vi "test Counter.vi"(8 "error in (no error)":errorcluster, 11 "TestCase in":refnum<class "Scan Engine Specialty Digital System Tests.lvclass">) -> (0 "error out":errorcluster, 3 "TestCase out":refnum<class "Scan Engine Specialty Digital System Tests.lvclass">)   [LabVIEW 2019, in "Scan Engine Specialty Digital System Tests.lvclass"]
uses:
  Scan Engine Specialty Digital System Tests.lvclass
  <vilib>/addons/_JKI Toolkits/VI Tester/TestCase.llb/TestCase.lvclass
  <vilib>/NI/VeriStand Custom Device Testing Tools/VeriStandTestUtilities/VeriStandTestUtilities.lvlib
  C:/Users/nitest/Desktop/Git 2019/niveristand-custom-device-testing-tools/VeriStandTestCase/VeriStandTestCase.lvclass
  C:/Program Files (x86)/National Instruments/LabVIEW 2019/vi.lib/addons/_JKI Toolkits/VI Tester/TestCase.llb/TestCase.lvclass
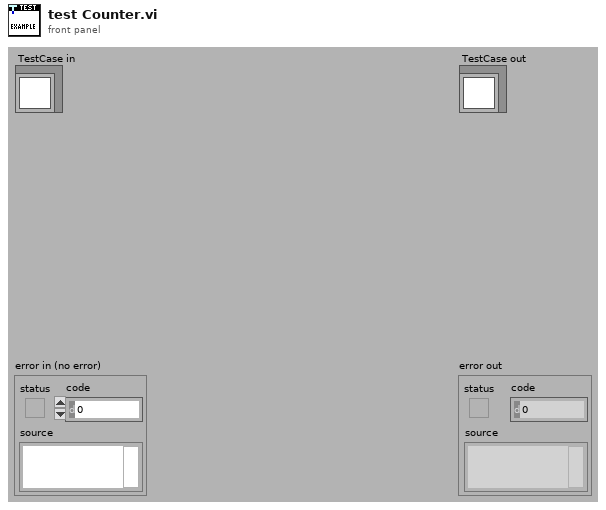
[diagram p1: front panel]
types:
  T1 = typedef "NI_VS Workspace ExecutionAPI.lvlib/WorkspaceAPI.ctl" = refnum<k24>
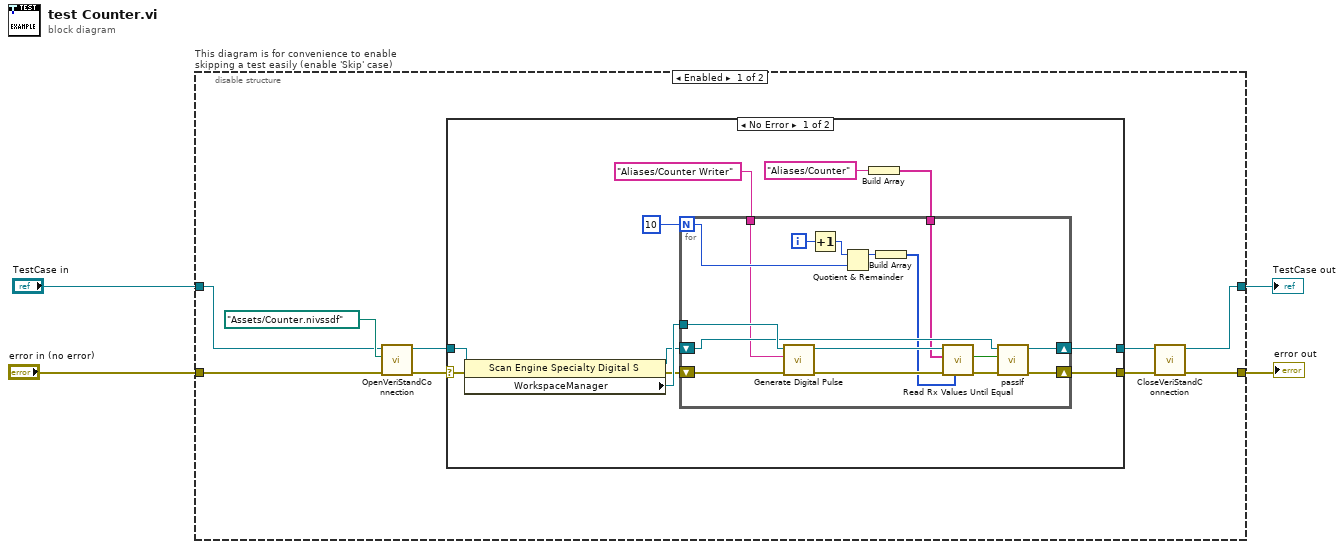
[diagram p0: block diagram]
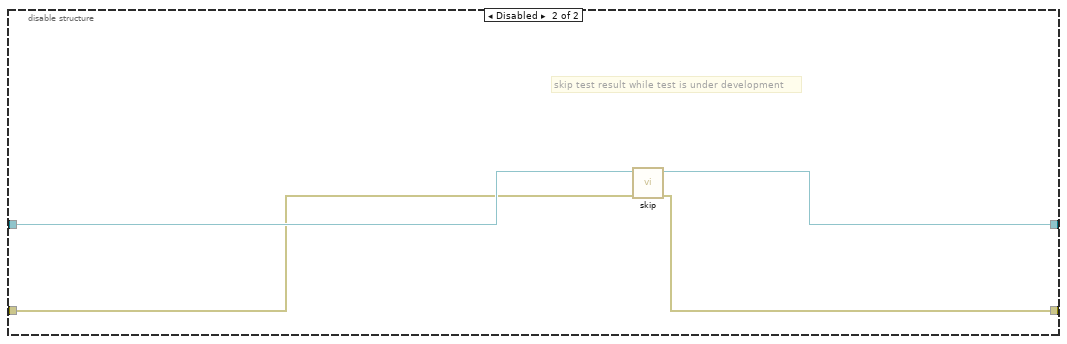
[diagram p3: hidden frame]
diagram:
  n1 = disable-structure "This diagram is for convenience to enable skipping a test easily (enable 'Skip' case)" shown="Enabled" {
    disable-tunnel: "TestCase in" -> [w9 w46]
    disable-tunnel: [w5 w44] -> w1
    disable-tunnel: [w7 w45] -> w3
    disable-tunnel: "error in (no error)" -> [w11 w43]
    frame Enabled {
      n2 = call-dynamic "OpenVeriStandConnection.vi"("error in (no error)"=w11, "System Definition File"=path "Assets/Counter.nivssdf", "VeriStand Test Case in"=w9) -> ("error out"=w12:errorcluster, "VeriStand Test Case out"=w10:refnum<class "Scan Engine Specialty Digital System Tests.lvclass">)  [unwired: 6 in, 1 out]
      n3 = case shown="No Error" w12 {
        selector: w12 -> [w17 w42]
        tunnel: [w21 w42] -> w8
        tunnel: [w15 w41] -> w6
        tunnel: w10 -> [w16 w41]
        frame No Error {
          n4 = property class="Scan Engine Specialty Digital S"(reference=w16, error in=w17) -> (reference out=w20:refnum<class "Scan Engine Specialty Digital System Tests.lvclass">, error out=w23:errorcluster, "WorkspaceManager"=w24:T1)
          n5 = Build Array("Aliases/Counter" ("Channel")) -> (w14:string[])
          n6 = for {
            N: 10 ("Terminal Count") -> [w30]
            tunnel: w24 -> [w40]
            shift-right: [w35] -> w21
            shift-left: w23 -> [w39]
            shift-right: [w32] -> w15
            shift-left: w20 -> [w33]
            tunnel: w14 -> [w28]
            tunnel: "Aliases/Counter Writer" ("Channel") -> [w29]
            i -> [w34]
            n7 = call "Generate Digital Pulse.vi"("error in (no error)"=w39, "Channel"=w29, "WorkspaceManager"=w40) -> ("error out"=w38:errorcluster, "Workspace Manager out"=w37:T1)  [unwired: 7 in]
            n8 = Increment(x=w34) -> (x+1=w31:i32)
            n9 = Quotient & Remainder(x=w31, y=w30) -> (x-y*floor(x/y)=w26:i32)  [unwired: 1 out]
            n10 = Build Array(w26) -> (w25:i32[])
            n11 = call <vilib>:"Read Rx Values Until Equal.vi"("expected values"=w25, "error in"=w38, "Rx aliases"=w28, "workspace manager in"=w37) -> ("error out"=w36:errorcluster, "values equal expected"=w27:bool)  [unwired: 5 in, 1 out]
            n12 = call-dynamic "passIf.vi"("error in (no error)"=w36, "pass"=w27, "TestCase in"=w33) -> ("error out"=w35:errorcluster, "TestCase out"=w32:refnum<class "Scan Engine Specialty Digital System Tests.lvclass">)  [unwired: 7 in]
          }
        }
        frame Error {
        }
      }
      n13 = call-dynamic "CloseVeriStandConnection.vi"("error in (no error)"=w8, "VeriStand Test Case in"=w6) -> ("error out"=w7:errorcluster, "VeriStand Test Case out"=w5:refnum<class "Scan Engine Specialty Digital System Tests.lvclass">)  [unwired: 8 in]
    }
    frame Disabled {
      # "skip test result while test is under development"
      n14 = call <vilib>:"skip.vi"("error in (no error)"=w43, "TestCase in"=w46) -> ("error out"=w45:errorcluster, "TestCase out"=w44:refnum<class "Scan Engine Specialty Digital System Tests.lvclass">)  [unwired: 8 in]
    }
  }
  "error out" <- w3
  "TestCase out" <- w1
